vi "rqp_Listen for Connections.vi"(7 "Caller in":refnum<class "Worker.lvclass">, 8 "error in":errorcluster, 9 "Data":T1, 11 "DS TCP Listener in":refnum<class "DS TCP Listener.lvclass">) -> (0 "error out":errorcluster, 3 "dup DS TCP Listener out":refnum<class "DS TCP Listener.lvclass">, 5 "dup Caller out":refnum<class "Worker.lvclass">)   [LabVIEW 2017, in "DS TCP Server.lvlib" / "DS TCP Listener.lvclass"]
doc: "This VI sends a <b>Public API Request</b> message to an MHL case of the Worker that owns this VI.\n---\nCreate a TCP listener, and listen continously on this port for incoming connections from Debug Clients."
uses:
  DS TCP Listener.lvclass
  C:/Program Files (x86)/National Instruments/LabVIEW 2017/vi.lib/addons/_Workers/Library/Classes/Worker/Worker.lvclass
  <vilib>/addons/_Workers/Library/Classes/Worker/Worker.lvclass
  rqp_Listen for Connections.ctl
  <vilib>/addons/_Workers/Library/Classes/Worker/Worker.lvclass/Worker.ctl
  <vilib>/addons/_Workers/Library/Classes/Message/Priority.ctl
  <vilib>/addons/_Workers/Library/Classes/Message/Enqueue Message to Queue.vi
  <vilib>/addons/_Workers/Library/Classes/Message/Message.lvclass
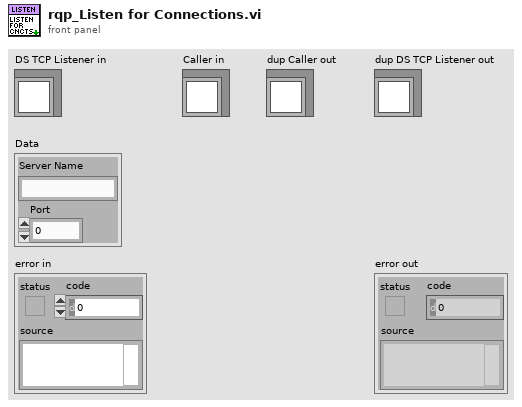
[diagram p1: front panel]
types:
  T1 = typedef "DS TCP Server.lvlib/DS TCP Listener.lvclass/rqp_Listen for Connections.ctl" = cluster{"Server Name":string, "Port":u16}
  T2 = typedef "Workers.lvlib/Message.lvclass/Priority.ctl" = enum16{"Low", "Normal", "High"}
  T3 = typedef "Workers.lvlib/Case Label.ctl" = string
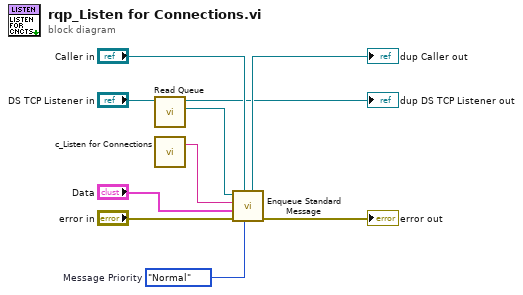
[diagram p0: block diagram]
diagram:
  w6 = Priority."Normal"  # Message Priority
  n1 = call <vilib>:"Read Queue.vi"("Worker_"="DS TCP Listener in") -> ("Message Queue out"=w3:refnum<class "Message Queue.lvclass">, "dup Worker_out"=→"dup DS TCP Listener out":refnum<class "DS TCP Listener.lvclass">)  [unwired: 9 in]
  n2 = call "c_Listen for Connections.vi"() -> ("Case Label"=w5:T3)  [unwired: 1 in]
  n3 = call-poly <vilib>:"Enqueue Standard Message.vi"("Priority (Normal)"=w6, "Worker"="Caller in", "error in"="error in", "Data"="Data", "Case Label"=w5, "Message Queue"=w3) -> ("error out"=→"error out":errorcluster, "dup Worker out"=→"dup Caller out":refnum<class "Worker.lvclass">)  [unwired: 3 in, 1 out]
